vi "closeFile.vi"(8 "error in (no error)":errorcluster, 11 "reference in":refnum<class "excelFile.lvclass">) -> (0 "error out":errorcluster, 3 "reference out":refnum<class "excelFile.lvclass">)   [LabVIEW 2015, in "excelFile.lvclass"]
uses:
  excelFile.lvclass
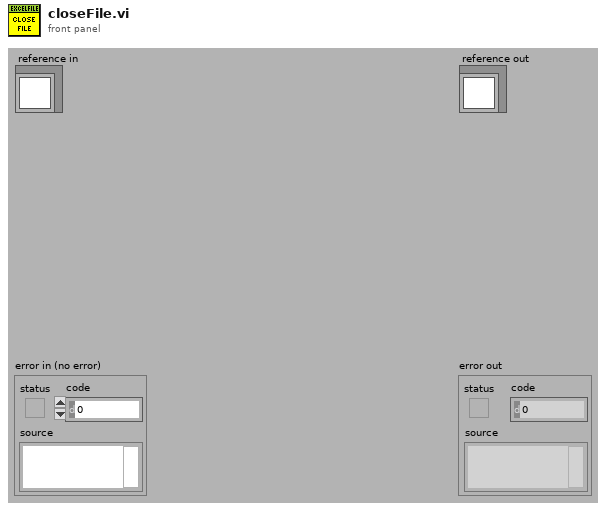
[diagram p1: front panel]
types:
  T1 = typedef "excelFile.lvclass/ObjectAttributesRef.ctl" = refnum<data-value>
  T2 = typedef "excelFile.lvclass/ObjectAttributes.ctl" = cluster{"MyAttribute":dbl, "path":string, "Refnum Excel":cluster{"Excel._Application":refnum<k7>, "Workbooks":refnum<k7>, "Open":refnum<k7>}, "data":string[][][], "save":bool, "fileType":T3, "rowsColor":u32[], "python_ref":refnum<class "python.lvclass">, "items_rows":i32[], "excel_range":i32[][], "TSR":cluster{"number":string, "TSR_path":path, "service_path":path, "email_to":string}, "excel_already_opened?":bool, "file_already_opened?":bool}
  T3 = typedef "excelFile.lvclass/fileType.ctl" = enum16{"devices", "items", "partsTracking", "TSR"}
  T4 = cluster{"Excel._Application":refnum<k7>, "Workbooks":refnum<k7>, "Open":refnum<k7>}
  T5 = cluster{"Excel._Application":refnum<k7>, "Workbooks":refnum<k7>}
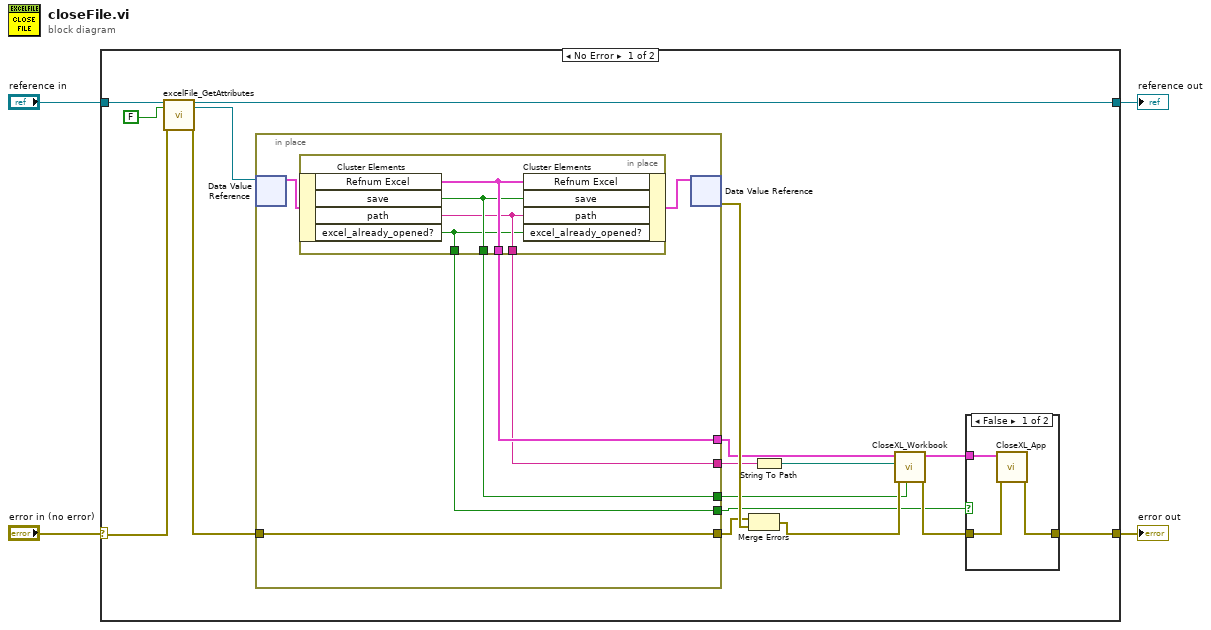
[diagram p0: block diagram]
diagram:
  n1 = case shown="No Error" "error in (no error)" {
    selector: "error in (no error)" -> [w17 w38]
    tunnel: [w8 w38] -> w3
    tunnel: [w15 w37] -> w1
    tunnel: "reference in" -> [w19 w37]
    frame No Error {
      n2 = call "excelFile_GetAttributes.vi"("reference in"=w19, "return data? (T)"=FALSE, "error in (no error)"=w17) -> ("reference out"=w15:refnum<class "excelFile.lvclass">, "attributes ref"=w14:T1, "error out"=w16:errorcluster)  [unwired: 13 in, 1 out]
      n3 = in-place {
        in-place-border: w16 -> [w30]
        in-place-border: [w30] -> w20
        in-place-border: [w29] -> w12
        in-place-border: [w28] -> w11
        in-place-border: [w27] -> w7
        in-place-border: [w26] -> w5
        n4 = in-place-dvr #1(w14) -> (w31:T2)  [unwired: 1 out]
        n5 = in-place {
          in-place-border: [w36] -> w29
          in-place-border: [w35] -> w28
          in-place-border: [w34] -> w27
          in-place-border: [w33] -> w26
          n6 = in-place-cluster #2(w31) -> ("Refnum Excel"=w36:T4, "save"=w35:bool, "path"=w34:string, "excel_already_opened?"=w33:bool)
          n7 = in-place-cluster #2("Refnum Excel"=w36, "save"=w35, "path"=w34, "excel_already_opened?"=w33) -> (w32:T2)
        }
        n8 = in-place-dvr #1(w32) -> (w21:errorcluster)  [unwired: 1 out]
      }
      n9 = Merge Errors(w20, w21) -> (w13:errorcluster)
      n10 = String To Path(string=w7) -> (path=w6:path)
      n11 = call <userlib>:"CloseXL_Workbook.vi"("Save? (F)"=w11, "error in (no error)"=w13, "path"=w6, "Refnum Cluster In"=w12) -> ("error out"=w9:errorcluster, "Refnum Cluster Out"=w10:T5)  [unwired: 6 in]
      n12 = case shown="False" w5 {
        tunnel: w10 -> [w24 _]
        tunnel: w9 -> [w23 w25]
        tunnel: [w22 w25] -> w8
        frame False {
          n13 = call <userlib>:"CloseXL_App.vi"("error in (no error)"=w23, "Refnum Cluster In"=w24) -> ("error out"=w22:errorcluster)  [unwired: 9 in]
        }
        frame True {
        }
      }
    }
    frame Error {
    }
  }
  "error out" <- w3
  "reference out" <- w1
